vi "mod_Modulate AM (SSB).vi"(0 "message signal":waveform(dbl)={"t0"=timestamp(0 s since 1904-01-01), "dt"=0.0, "Y"=[]}, 2 "pilot tone":T1={"frequency (Hz)"=0.0, "amplitude"=1.0}, 5 "AM SSB-VSB parameters":T2={"modulation index"=1.0, "side-band"=enum."Lower sideband", "suppress carrier ?"=FALSE} {"modulation index" format="%.2f"}, 7 "hilbert filter":T3={"taps"=81, "design"=enum."Windowed Hilbert Transformer"}, 9 "peak message amplitude":dbl=1.0, 11 "error in (no error)":errorcluster, 13 "reset? (T)":bool=TRUE) -> (4 "output complex waveform":T4 {"Y" format="%.3f"; "dt" format="%^.2e"; "t0" format="%.4f"}, 15 "error out":errorcluster)   [LabVIEW 2020, in "niAMT.lvlib"]
uses:
  <vilib>/addons/Modulation/niAMT.lvlib
  <vilib>/addons/Modulation/Analog/controls/Complex Data Waveform.ctl
  <vilib>/addons/Modulation/Analog/controls/mod_Hilbert filter.ctl
  <vilib>/addons/Modulation/Analog/controls/mod_AM parameters.ctl
  <vilib>/addons/Modulation/Analog/controls/mod_AM pilot tone.ctl
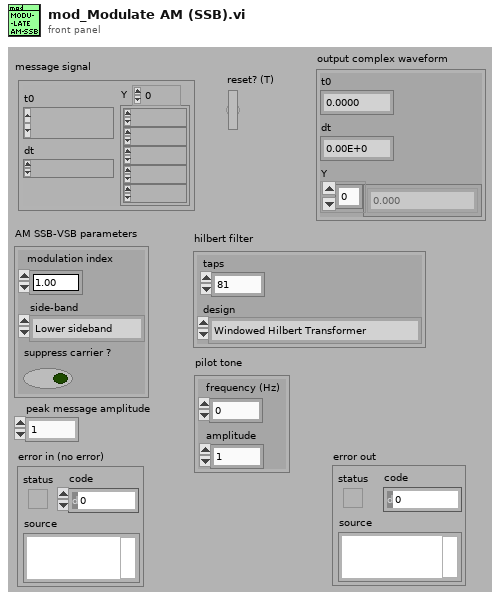
[diagram p1: front panel]
types:
  T1 = typedef "niAMT.lvlib/mod_AM pilot tone.ctl" = cluster{"frequency (Hz)":dbl, "amplitude":dbl}
  T2 = typedef "niAMT.lvlib/mod_AM parameters.ctl" = cluster{"modulation index":dbl, "side-band":enum16{"Lower sideband", "Upper sideband"}, "suppress carrier ?":bool}
  T3 = typedef "niAMT.lvlib/mod_Hilbert filter.ctl" = cluster{"taps":i32, "design":enum16{"Windowed Hilbert Transformer", "Equiripple Hilbert transformer"}}
  T4 = typedef "niAMT.lvlib/Complex Data Waveform.ctl" = cluster{"t0":dbl, "dt":dbl, "Y":cdb[]}
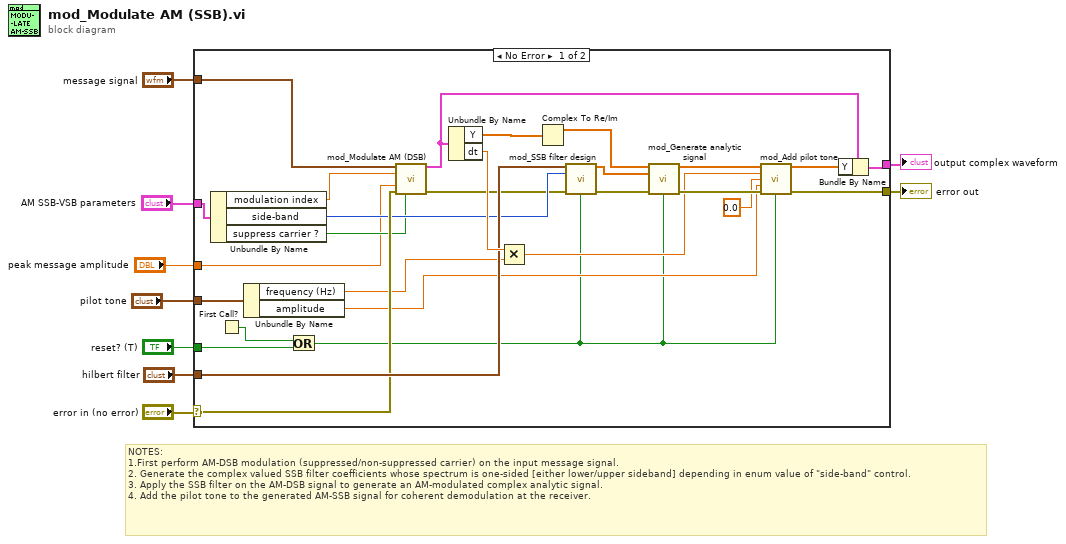
[diagram p0: block diagram]
diagram:
  # "NOTES:\n1.First perform AM-DSB modulation (suppressed/non-suppressed carrier) on the input message signal.\n2. Generate the complex valued SSB filter coefficients whose spectrum is one-sided [either lower/upper sideband] depending in enum value of \"side-band\" control.\n3. Apply the SSB filter on the AM-DSB signal to generate an AM-modulated complex analytic signal.\n4. Add the pilot tone to the generated AM-SSB signal for coherent demodulation at the receiver."
  n1 = case shown="No Error" "error in (no error)" {
    selector: "error in (no error)" -> [w22 w38]
    tunnel: [w32 w38] -> w8
    tunnel: [w28 _] -> w7
    tunnel: "message signal" -> [w25 _]
    tunnel: "reset? (T)" -> [w24 _]
    tunnel: "hilbert filter" -> [w23 _]
    tunnel: "AM SSB-VSB parameters" -> [w19 _]
    tunnel: "pilot tone" -> [w14 _]
    tunnel: "peak message amplitude" -> [w10 _]
    frame No Error {
      n2 = Unbundle By Name(w19) -> ("modulation index"=w18:dbl, "side-band"=w17:enum16{"Lower sideband", "Upper sideband"}, "suppress carrier ?"=w16:bool)
      n3 = First Call?() -> (First Call?: T/F=w26:bool)
      n4 = Unbundle By Name(w14) -> ("frequency (Hz)"=w13:dbl, "amplitude"=w12:dbl)
      n5 = Or(x=w26, y=w24) -> (x .or. y?=w11:bool)
      n6 = call <vilib>:"mod_Modulate AM (DSB).vi"("message signal"=w25, "modulation index"=w18, "peak message amplitude"=w10, "error in (no error)"=w22, "suppress carrier ?"=w16) -> ("AM modulated waveform"=w37:cluster{"t0":dbl, "dt":dbl, "Y":cdb[]}, "error out"=w15:errorcluster)  [unwired: 2 in, 7 out]
      n7 = Unbundle By Name(w37) -> ("Y"=w36:cdb[], "dt"=w30:dbl)
      n8 = Multiply(x=w30, y=w13) -> (x*y=w29:dbl)
      n9 = Complex To Re/Im(x + iy=w36) -> (x=w35:dbl[])  [unwired: 1 out]
      n10 = call <vilib>:"mod_SSB filter design.vi"("hilbert filter"=w23, "side-band"=w17, "error in (no error)"=w15, "reset? (T)"=w11) -> ("AM-SSB filter taps"=w21:cdb[], "error out"=w20:errorcluster)  [unwired: 1 in, 9 out]
      n11 = call <vilib>:"mod_Generate analytic signal.vi"("m(t)"=w35, "filter taps"=w21, "error in (no error)"=w20, "reset? (T)"=w11) -> ("analytic signal"=w34:cdb[], "error out"=w33:errorcluster)  [unwired: 10 out]
      n12 = call <vilib>:"mod_Add pilot tone.vi"("input"=w34, "pilot tone frequency (normalized)"=w29, "starting phase (radians)"=0.0, "pilot tone amplitude"=w12, "error in (no error)"=w33, "reset? (T)"=w11) -> ("input+pilot tone"=w31:cdb[], "error out"=w32:errorcluster)  [unwired: 8 out]
      n13 = Bundle By Name(cluster=w37, "Y"=w31) -> (w28:cluster{"t0":dbl, "dt":dbl, "Y":cdb[]})
    }
    frame Error {
    }
  }
  "error out" <- w8
  "output complex waveform" <- w7
